vi "Special 1 Step 2 (SubVI).vi"(0 "Ldist":dbl, 5 "Rdist":dbl, 7 "Tside":dbl, 9 "lbrc":dbl, 11 "rblc":dbl) -> (4 "aLB":dbl, 6 "aRB":dbl, 8 "aLB1":dbl, 10 "aRB1":dbl)   [LabVIEW 2015]
uses:
  <vilib>/express/express arith-compare/Formula/XNode/ExpressFormulaBlockNode.xnode
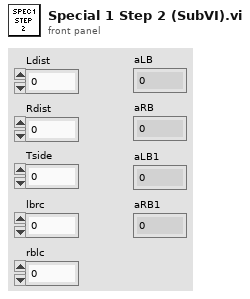
[diagram p1: front panel]
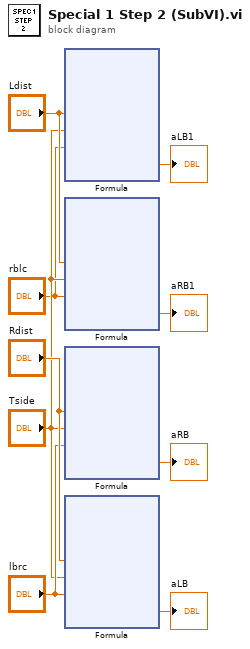
[diagram p0: block diagram]
diagram:
  n1 = xnode "Formula"("Ldist"="Ldist", "Tside"="Tside", "rblc"="rblc") -> ("Result"=→"aLB1":dbl)  [unwired: 1 in, 1 out]
  n2 = xnode "Formula"("Ldist"="Ldist", "Tside"="Tside", "rblc"="rblc") -> ("Result"=→"aRB1":dbl)  [unwired: 1 in, 1 out]
  n3 = xnode "Formula"("Rdist"="Rdist", "Tside"="Tside", "lbrc"="lbrc") -> ("Result"=→"aRB":dbl)  [unwired: 1 in, 1 out]
  n4 = xnode "Formula"("Rdist"="Rdist", "Tside"="Tside", "lbrc"="lbrc") -> ("Result"=→"aLB":dbl)  [unwired: 1 in, 1 out]
